vi "global_variable_STOP.vi"() -> ()   [LabVIEW 2022 SP3]
panel:
  in  "GLOBAL STOP":bool
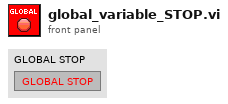
[diagram p1: front panel]
diagram:
